vi "_Set Fp Cluster Autosizing Property.vi"(8 "error in (no error)":errorcluster, 10 "type":T1(ring), 11 "SelList[]":refnum<vi>[](array[refnum])) -> (0 "error out":errorcluster, 3 "Changed":bool)   [LabVIEW 2017, in "Cluster AutoSizing.lvlib"]
uses:
  Cluster AutoSizing.lvlib
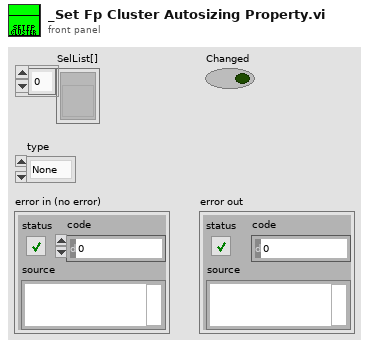
[diagram p1: front panel]
types:
  T1 = enum16{"None", "Size to Fit", "Arrange Horizontally", "Arrange Veritcally"}
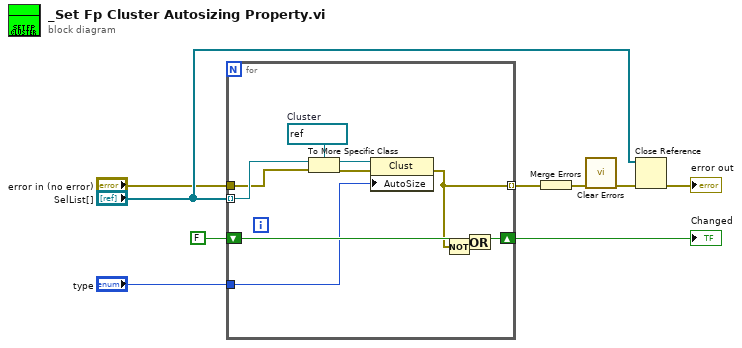
[diagram p0: block diagram]
diagram:
  n1 = for {
    shift-right: [w18] -> w3
    shift-left: FALSE -> [w19]
    tunnel: "SelList[]" -> [w17] mode=indexing
    tunnel: "error in (no error)" -> [w14]
    tunnel: [w11] -> w4 mode=indexing
    tunnel: "type" -> [w13]
    w15 = refnum<vi> refnum  # Cluster
    n2 = To More Specific Class(target class=w15, reference=w17, error in=w14) -> (specific class reference=w16:refnum<vi>, error out=w12:errorcluster)
    n3 = property class="Clust"(reference=w16, error in=w12, "AutoSize"=w13) -> (error out=w11:errorcluster)  [unwired: 1 out]
    n4 = Not(x=w11) -> (.not. x?=w10:bool)
    n5 = Or(x=w19, y=w10) -> (x .or. y?=w18:bool)
  }
  "Changed" <- w3
  n6 = Merge Errors(w4) -> (w6:errorcluster)
  n7 = call <vilib>:"Clear Errors.vi"("error in (no error)"=w6) -> ("error out"=w7:errorcluster)  [unwired: 5 in, 1 out]
  n8 = Close Reference(reference="SelList[]", error in (no error)=w7) -> (error out=→"error out":errorcluster)
